vi "Get CEID Data.vi"(8 "error in (no error)":errorcluster, 11 "07-Event Report From Equipment in":refnum<class "07-Event Report From Equipment.lvclass">) -> (0 "error out":errorcluster, 1 "OK?":bool, 2 "S6F11":T1, 3 "07-Event Report From Equipment out":refnum<class "07-Event Report From Equipment.lvclass">)   [LabVIEW 2020, in "SECS Scenarios.lvlib" / "07-Event Report From Equipment.lvclass"]
uses:
  07-Event Report From Equipment.lvclass
  SECS Communication/S6 Message Class/S6F11.ctl
  07-Event Report From Equipment.lvclass/07-Event Report From Equipment.ctl
  SECS Communication/SECS-II Class/Format Code.ctl
  SECS Communication/SECS Data Class/Get RPTID Data.vi
  SECS Communication/SECS Data Class/Get SVID Data.vi
  SECS Communication/SECS Data Class/Get ECID Data.vi
  SECS Communication/SECS Data Class/Get ALID Data.vi
  SECS Communication/SECS Data Class/SECS Data Class.lvclass
  SECS Communication/SECS-II Class/SECS-II Class.lvclass
  SECS Communication/S6 Message Class/S6 Message Class.lvclass
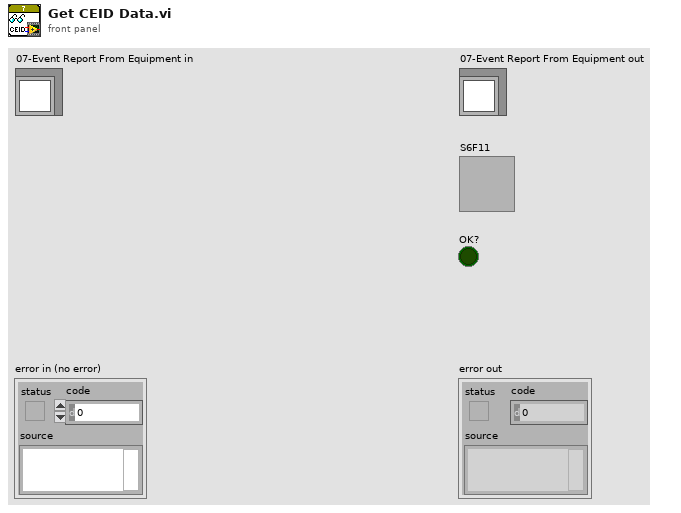
[diagram p1: front panel]
types:
  T1 = typedef "SECS Communication.lvlib/S6 Message Class.lvclass/S6F11.ctl" = cluster{"DATAID":u32, "CEID":u32, "Report Data":cluster{"RPTID":u32, "Value":cluster{"Format Code":T2, "Value":variant}[]}[]}
  T2 = typedef "SECS Communication.lvlib/SECS-II Class.lvclass/Format Code.ctl" = enum16{"L", "A", "B", "Boolean", "J", "I1", "I2", "I4", "I8", "U1", "U2", "U4", "U8", "F4", "F8", "Char"}
  T3 = typedef "SECS Communication.lvlib/SECS Data Class.lvclass/CEID Data.ctl" = cluster{"Enable":bool, "CEID":u32, "Name":string, "Description":string, "RPTID":u32[], "Dynamic":bool}
  T4 = typedef "SECS Communication.lvlib/SECS Data Class.lvclass/RPTID Data.ctl" = cluster{"RPTID":u32, "Report Information":string[], "Dynamic":bool}
  T5 = typedef "SECS Communication.lvlib/SECS Data Class.lvclass/SVID Data.ctl" = cluster{"SVID":u32, "Name":string, "Description":string, "Format Code":T2, "Unit":string, "Source":string, "Data":variant}
  T6 = typedef "SECS Communication.lvlib/SECS Data Class.lvclass/ECID Data.ctl" = cluster{"ECID":u32, "Name":string, "Description":string, "Format Code":T2, "Unit":string, "Max":dbl, "Min":dbl, "Default":string, "Source":string, "Data":variant}
  T7 = typedef "SECS Communication.lvlib/SECS Data Class.lvclass/ALID Data.ctl" = cluster{"Enable":bool, "ALID":u32, "Name":string, "Description":string, "Source":string, "Status":enum16{"Null", "Normal", "Abnormal", "Warning"}}
  T8 = cluster{"RPTID":u32, cluster{"Format Code":T2, "Variant":variant}[]}
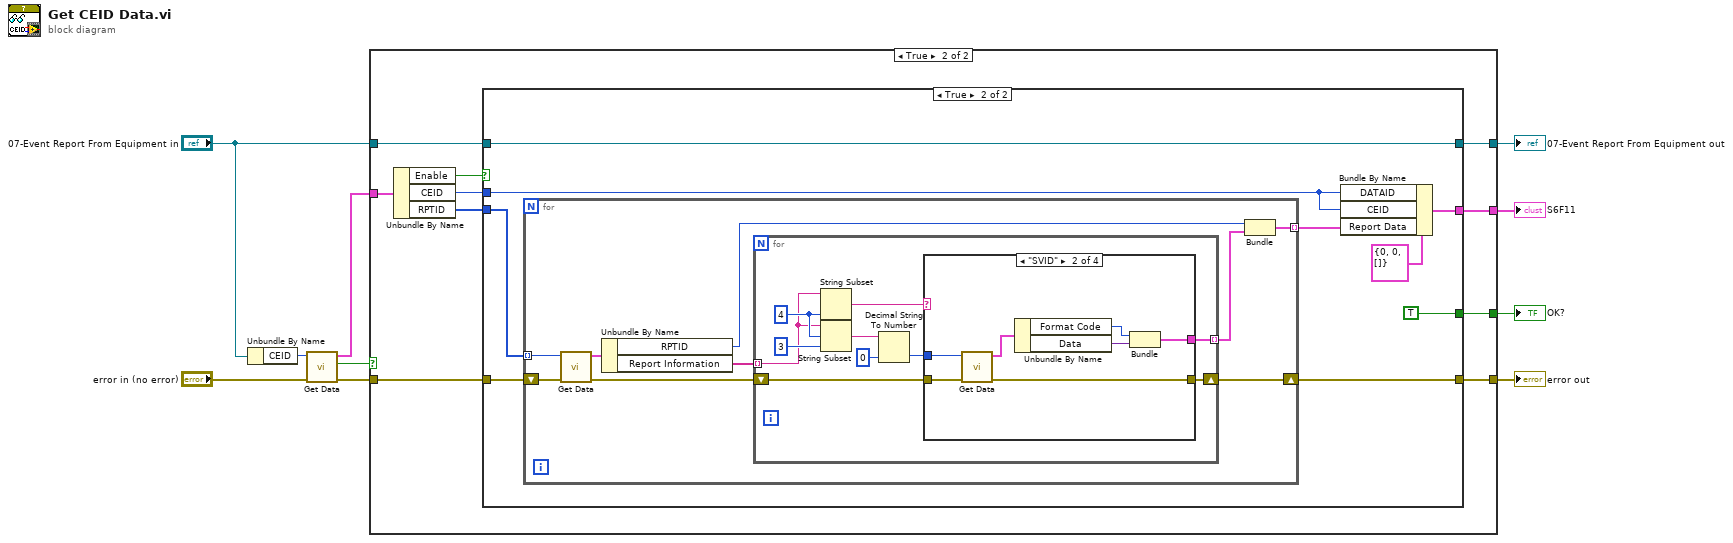
[diagram p0: block diagram]
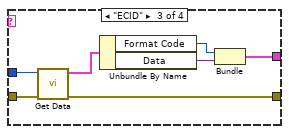
[diagram p5: hidden frame]
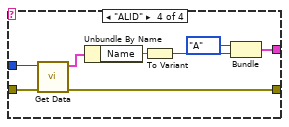
[diagram p6: hidden frame]
diagram:
  n1 = Unbundle By Name("07-Event Report From Equipment in") -> ("CEID"=w10:u32)
  n2 = call-poly "Get Data.vi"("error in"="error in (no error)", "CEID"=w10) -> ("error out"=w9:errorcluster, "Find?"=w8:bool, "CEID Data"=w7:T3)  [unwired: 7 in]
  n3 = case shown="True" w8 {
    tunnel: w9 -> [w11 w21]
    tunnel: w7 -> [_ w22]
    tunnel: "07-Event Report From Equipment in" -> [w12 w19]
    tunnel: [w12 w17] -> w3
    tunnel: [w11 w15] -> w4
    tunnel: [_ w14] -> w1
    tunnel: [_ w13] -> w2
    frame False {
    }
    frame True {
      n4 = Unbundle By Name(w22) -> ("Enable"=w16:bool, "CEID"=w18:u32, "RPTID"=w20:u32[])
      n5 = case shown="True" w16 {
        tunnel: w21 -> [w23 w33]
        tunnel: w20 -> [_ w27]
        tunnel: w19 -> [w24 w30]
        tunnel: w18 -> [_ w31]
        tunnel: [w24 w30] -> w17
        tunnel: [_ w29] -> w13
        tunnel: [w23 w28] -> w15
        tunnel: [_ TRUE] -> w14
        frame False {
        }
        frame True {
          n6 = for {
            shift-right: [w38] -> w28
            shift-left: w33 -> [w42]
            tunnel: w27 -> [w37] mode=indexing
            tunnel: [w34] -> w26 mode=indexing
            n7 = call-poly "Get Data.vi"("error in"=w42, "RPTID"=w37) -> ("error out"=w40:errorcluster, "RPTID Data"=w41:T4)  [unwired: 7 in, 1 out]
            n8 = Unbundle By Name(w41) -> ("RPTID"=w35:u32, "Report Information"=w39:string[])
            n9 = for {
              shift-right: [w44] -> w38
              shift-left: w40 -> [w46]
              tunnel: w39 -> [w43] mode=indexing
              tunnel: [w45] -> w36 mode=indexing
              w52 = 4 ("length (rest)")
              n10 = String Subset(string=w43, length (rest)=w52) -> (substring=w48:string)  [unwired: 1 in]
              n11 = String Subset(string=w43, offset (0)=w52, length (rest)=3 ("length (rest)")) -> (substring=w50:string)
              n12 = Decimal String To Number(string=w50, default (0L)=u32 0 ("default (0 I32)")) -> (number=w47:u32)  [unwired: 1 in, 1 out]
              n13 = case shown="\"SVID\"" w48 {
                tunnel: w47 -> [_ w59 w66 w71]
                tunnel: w46 -> [w53 w60 w67 w72]
                tunnel: [_ w55 w62 w75] -> w45
                tunnel: [w53 w54 w61 w70] -> w44
                frame Default {
                }
                frame "SVID" {
                  n14 = call-poly "Get Data.vi"("error in"=w60, "SVID"=w59) -> ("error out"=w54:errorcluster, "SVID Data"=w58:T5)  [unwired: 7 in, 1 out]
                  n15 = Unbundle By Name(w58) -> ("Format Code"=w56:T2, "Data"=w57:variant)
                  n16 = Bundle("Format Code"=w56, "Data"=w57) -> (w55:cluster{"Format Code":T2, "Data":variant})  [unwired: 1 in]
                }
                frame "ECID" {
                  n17 = call-poly "Get Data.vi"("error in"=w67, "ECID"=w66) -> ("error out"=w61:errorcluster, "ECID Data"=w65:T6)  [unwired: 7 in, 1 out]
                  n18 = Unbundle By Name(w65) -> ("Format Code"=w63:T2, "Data"=w64:variant)
                  n19 = Bundle("Format Code"=w63, "Data"=w64) -> (w62:cluster{"Format Code":T2, "Data":variant})  [unwired: 1 in]
                }
                frame "ALID" {
                  n20 = call-poly "Get Data.vi"("error in"=w72, "ALID"=w71) -> ("error out"=w70:errorcluster, "ALID Data"=w69:T7)  [unwired: 7 in, 1 out]
                  n21 = Unbundle By Name(w69) -> ("Name"=w68:string)
                  n22 = To Variant(anything=w68) -> (Variant=w73:variant)
                  n23 = Bundle("Format Code"=Format_Code."A", "Variant"=w73) -> (w75:cluster{"Format Code":T2, "Variant":variant})  [unwired: 1 in]
                }
              }
            }
            n24 = Bundle("RPTID"=w35, w36) -> (w34:T8)  [unwired: 1 in]
          }
          n25 = Bundle By Name(cluster=T1 {"DATAID"=0, "CEID"=0, "Report Data"=[]} ("S6F11"), "DATAID"=w31, "CEID"=w31, "Report Data"=w26) -> (w29:T1)
        }
      }
    }
  }
  "error out" <- w4
  "07-Event Report From Equipment out" <- w3
  "S6F11" <- w2
  "OK?" <- w1
